vi "Cleanup Client.vi"(8 "error in (no error)":errorcluster, 11 "TCPMessaging in":refnum<class "TCPMessaging.lvclass">) -> (0 "error out":errorcluster)   [LabVIEW 2020, in "Vecto.lvlib" / "TCPMessaging.lvclass"]
uses:
  TCPMessaging.lvclass
  TCPMessaging.lvclass/TCPMessaging.ctl
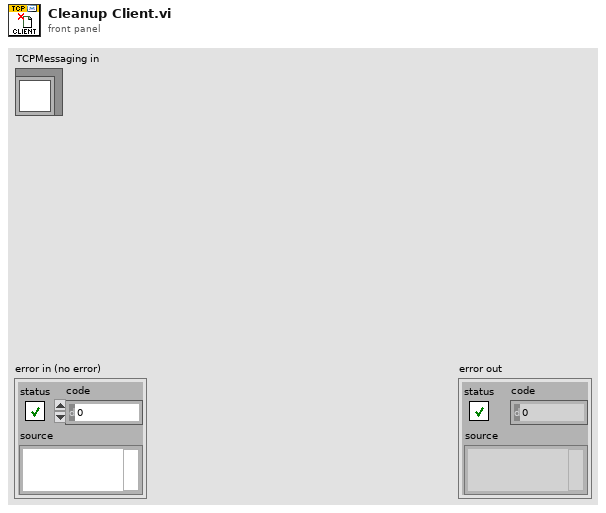
[diagram p1: front panel]
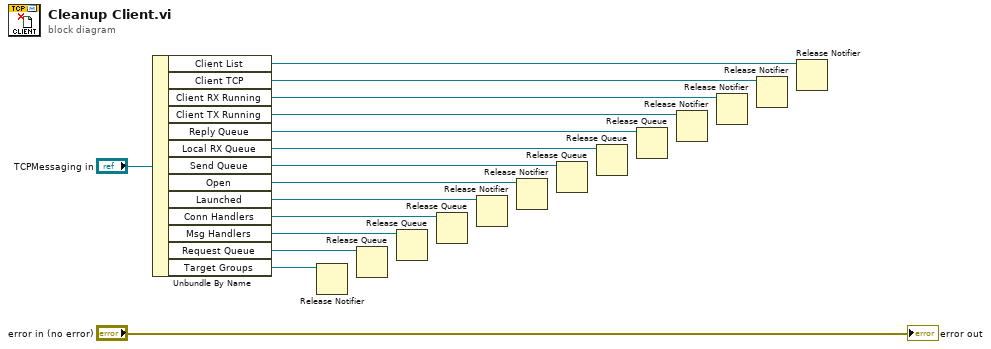
[diagram p0: block diagram]
diagram:
  n1 = Unbundle By Name("TCPMessaging in") -> ("Client List"=w1:refnum<notifier>, "Client TCP"=w2:refnum<notifier>, "Client RX Running"=w3:refnum<notifier>, "Client TX Running"=w4:refnum<notifier>, "Reply Queue"=w11:refnum<queue>, "Local RX Queue"=w12:refnum<queue>, "Send Queue"=w13:refnum<queue>, "Open"=w14:refnum<notifier>, "Launched"=w10:refnum<notifier>, "Conn Handlers"=w9:refnum<queue>, "Msg Handlers"=w8:refnum<queue>, "Request Queue"=w7:refnum<queue>, "Target Groups"=w6:refnum<notifier>)
  n2 = Release Notifier(notifier=w6) -> ()  [unwired: 2 in, 3 out]
  n3 = Release Queue(queue=w7) -> ()  [unwired: 2 in, 3 out]
  n4 = Release Queue(queue=w8) -> ()  [unwired: 2 in, 3 out]
  n5 = Release Queue(queue=w9) -> ()  [unwired: 2 in, 3 out]
  n6 = Release Notifier(notifier=w10) -> ()  [unwired: 2 in, 3 out]
  n7 = Release Notifier(notifier=w14) -> ()  [unwired: 2 in, 3 out]
  n8 = Release Queue(queue=w13) -> ()  [unwired: 2 in, 3 out]
  n9 = Release Queue(queue=w12) -> ()  [unwired: 2 in, 3 out]
  n10 = Release Queue(queue=w11) -> ()  [unwired: 2 in, 3 out]
  n11 = Release Notifier(notifier=w4) -> ()  [unwired: 2 in, 3 out]
  n12 = Release Notifier(notifier=w3) -> ()  [unwired: 2 in, 3 out]
  n13 = Release Notifier(notifier=w2) -> ()  [unwired: 2 in, 3 out]
  n14 = Release Notifier(notifier=w1) -> ()  [unwired: 2 in, 3 out]
  "error out" <- "error in (no error)"
